vi "Qudi_ROI_multicolour_scan_Kinetix.vi"(3 "N Z positions":i32) -> ()   [LabVIEW 2015]
uses:
  <vilib>/rvi/Analysis/control/PID/Typedef/niFpgaPID_PIGains.ctl
  <vilib>/Platform/TimedLoop/XDataNode/timing_clust.ctl
  <vilib>/Platform/TimedLoop/XDataNode/nitl_modes.ctl
  <vilib>/Platform/TimedLoop/XDataNode/wakeup.ctl
  <vilib>/rvi/FXPMathLib/basic elements/FxpIntAccumulator/subVIs/nifxpmath_IntAccumulator_SimConfig.ctl
  <vilib>/rvi/Emulation/niFpgaGetClockAttributes.vi
  <vilib>/rvi/Emulation/niFpgaSctlEmulationGetInTimedLoop.vi
  <vilib>/rvi/Emulation/niFpgaEmulationReportErrorSimple.vi
  <vilib>/rvi/Emulation/niFpgaProcessEmulError.vi
  <vilib>/rvi/eio/common/nirviEmuTemplateMethod_errors.vi
  <vilib>/rvi/Analysis/common/codeGenErrors/XNode/niFpgaXNodeCodeGenErrorHandle.vi
  <vilib>/rvi/Emulation/niFpgaCriticalErrorInLSC.vi
  <vilib>/rvi/FXPMathLib/basic elements/FxpIntAccumulator/simVIs/DllFxpIntAccumulator_sub.vi
  <vilib>/rvi/Analysis/control/PID/SubVIs/niFpgaPID_PIWrapper.vi
  <vilib>/eio/EIONode/EIONode.xnode
  <vilib>/rvi/Analysis/measure/dc-rms/XNode/niFpgaDC-RMS.xnode
  <vilib>/Platform/TimedLoop/XDataNode/XDataNode.xnode
  <vilib>/rvi/FXPMathLib/basic elements/FxpIntAccumulator/XNode/nifxpmath_IntAccumulator.xnode
  <vilib>/rvi/FXPMathLib/FxpMul/XNode/nifxpmath_Multiplier.xnode
  <vilib>/Platform/TimedLoop/XDataNode/XDNodeRunTimeDep.lvlib
  <vilib>/rvi/FXPMathLib/sim/FxpSim.dll
panel:
  out "duration_ms":u32
  out "X":i16
  out "Y":i16
  out "Sum":i16
  out "counter":u32
  out "output":i16
  in  "reset":bool
  in  "reset_counter":bool
  in  "autofocus":bool
  in  "setpoint":i16
  in  "P":i16
  in  "I":i16
  in  "ref_axis":bool
  in  "integration_time_us":u32=100 caption="Count(uSec)"
  in  "exposure_time_ms":u16
  in  "stop":bool
  out "Images acquired":i32
  in  "Laser lines":i32[](array[numeric])=[0, 0, 0, 0, 0, 0, 0, 0, 0, 0]
  in  "N laser lines":i32
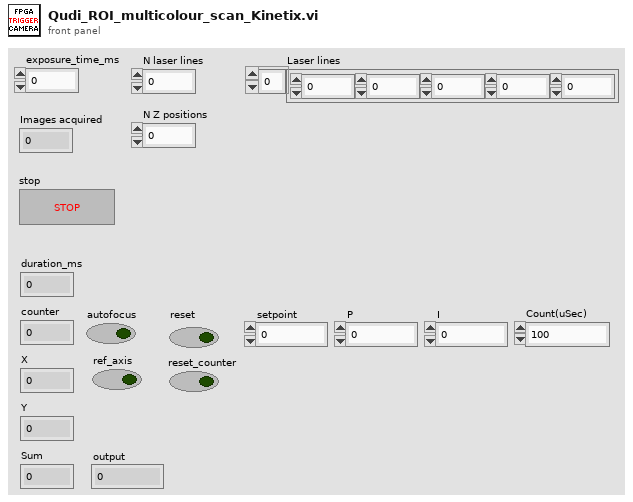
[diagram p1: front panel]
types:
  T1 = typedef "niFpgaPID_PIGains.ctl" = cluster{"proportional gain":sgl, "integral gain":sgl}
  T2 = typedef "XDNodeRunTimeDep.lvlib/timing_clust.ctl" = cluster{"Expected End [f-1]":u64, "Actual End [f-1]":u64, "Finished Late? [f-1]":bool, "Expected End [i-1]":u64, "Actual End [i-1]":u64, "Finished Late? [i-1]":bool, "Expected Start [i]":u64, "Actual Start [i]":u64, "Expected Start [f]":u64, "Actual Start [f]":u64, "Source Name":string, "Structure Name":string, "Period":i64, "Deadline":i64, "Offset":i64, "Start":i64, "Priority":i32, "Timeout":i32, "Mode":T3, "Wakeup Reason":T4, "Error":errorcluster, "Source Type":string, "Secondary Source Type":string, "Global End Time":u64, "Global Start Time":u64, "Frame Duration":u64, "Iteration Duration":u64, "Assigned CPU":i32, "I/O Scan Engine Mode":u32}
  T3 = typedef "XDNodeRunTimeDep.lvlib/nitl_modes.ctl" = enum32{"No Change", "Process missed periods, maintain original phase", "Discard missed periods, maintain original phase", "Process missed periods, ignore original phase", "Discard missed periods, ignore original phase"}
  T4 = typedef "XDNodeRunTimeDep.lvlib/wakeup.ctl" = enum32{"Normal", "Aborted", "Asynchronous wakeup", "Timing source error", "Timed loop error", "Timeout"}
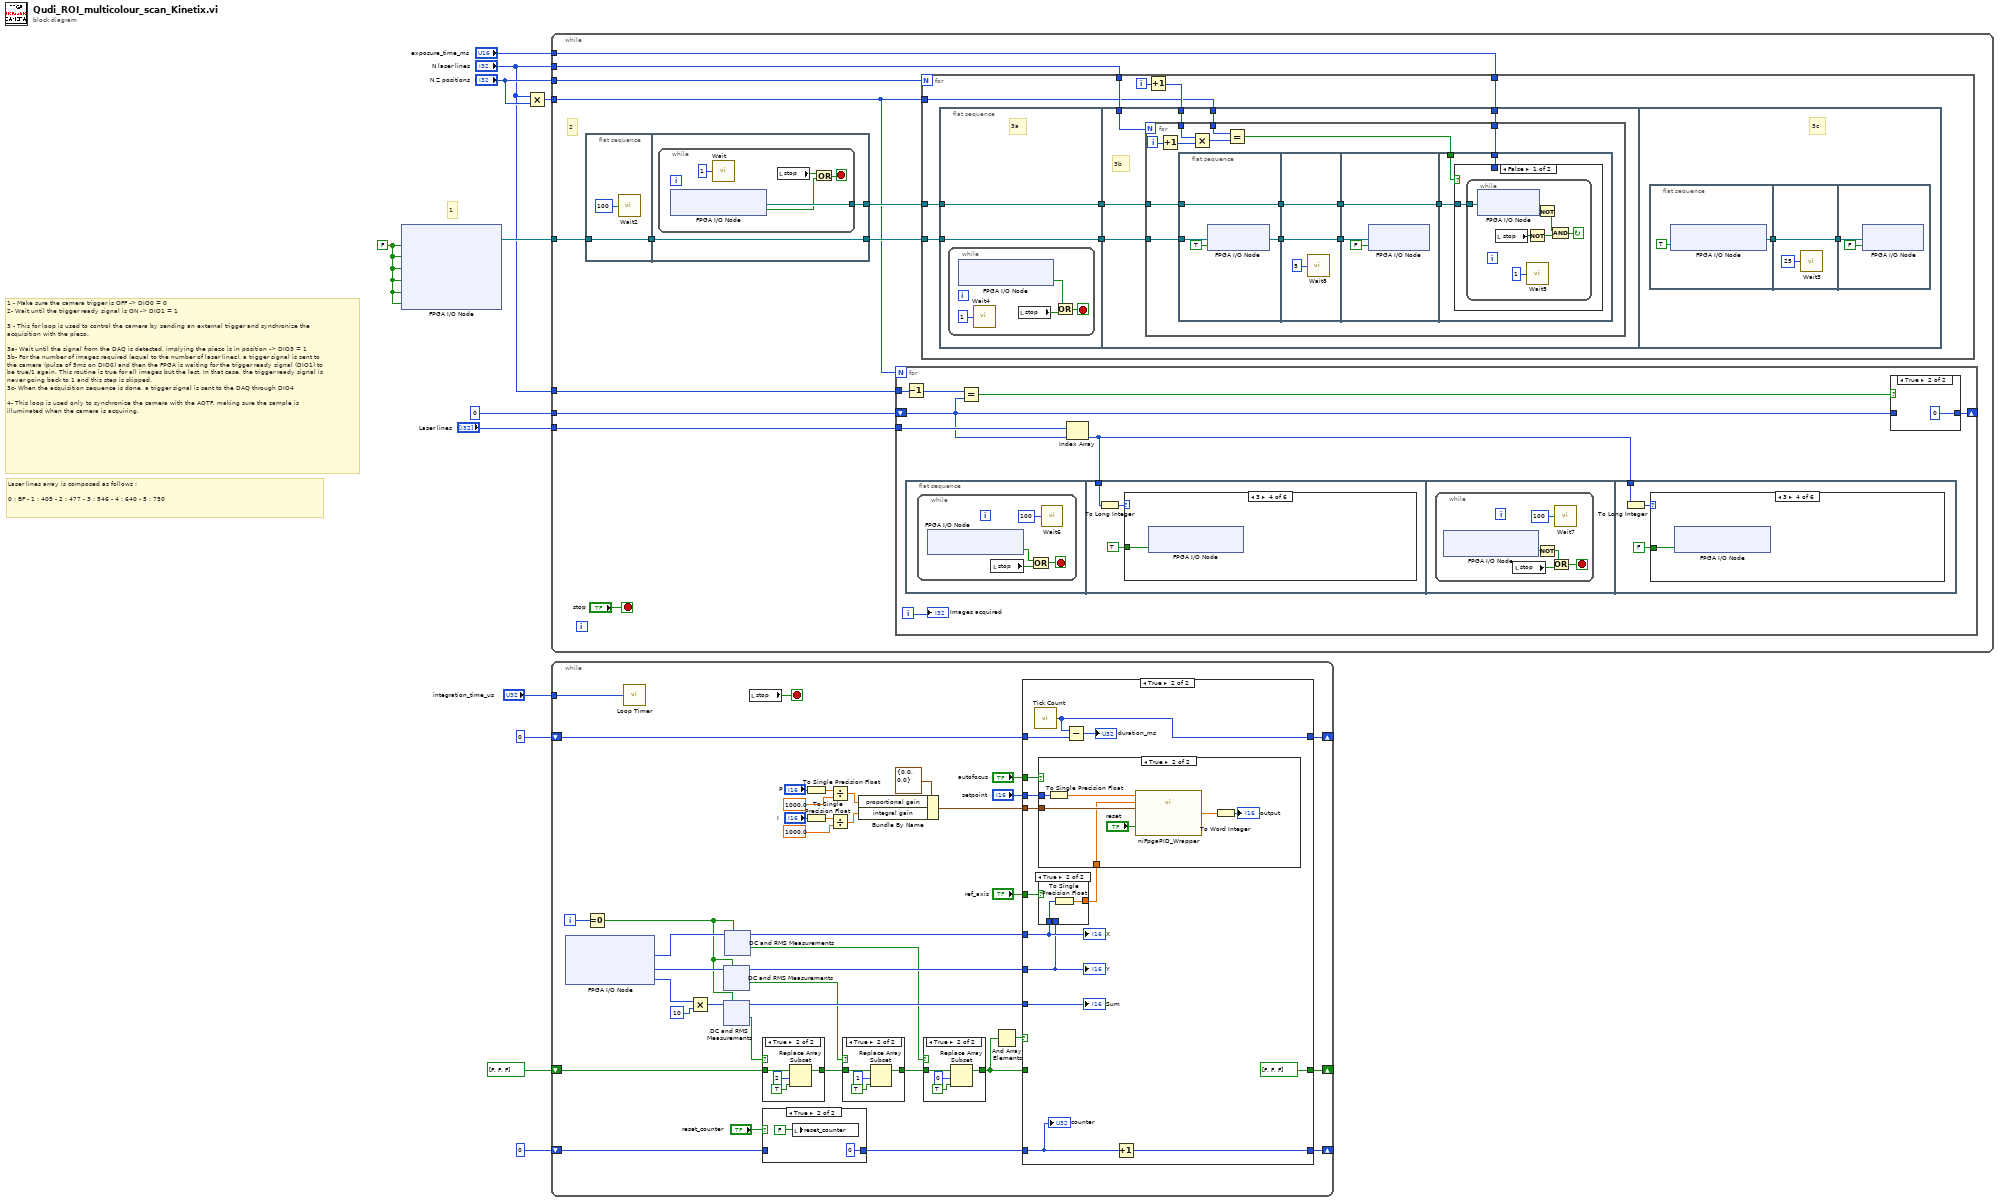
[diagram p0: block diagram]
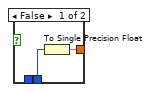
[diagram p7: hidden frame]
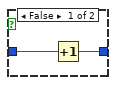
[diagram p9: hidden frame]
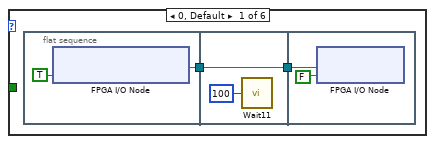
[diagram p10: hidden frame]
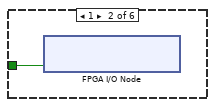
[diagram p11: hidden frame]
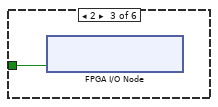
[diagram p12: hidden frame]
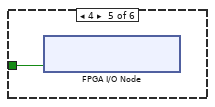
[diagram p13: hidden frame]
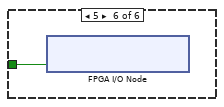
[diagram p14: hidden frame]
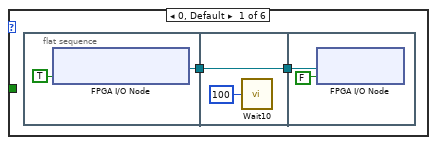
[diagram p15: hidden frame]
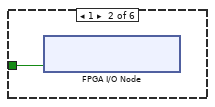
[diagram p16: hidden frame]
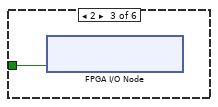
[diagram p17: hidden frame]
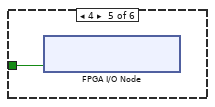
[diagram p18: hidden frame]
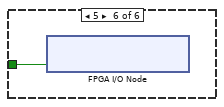
[diagram p19: hidden frame]
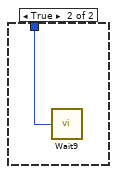
[diagram p20: hidden frame]
diagram:
  w5 = FALSE ("Connector0/DIO0")
  # "Laser lines array is composed as follows :\n\n0 : BF - 1 : 405 - 2 : 477 - 3 : 546 - 4 : 640 - 5 : 750"
  # "1"
  # "1 - Make sure the camera trigger is OFF -> DIO0 = 0\n2- Wait until the trigger ready signal is ON -> DIO1 = 1\n\n3 - This for loop is used to control the camera by sending an external trigger and synchronize the acquisition with the piezo.\n\n3a- Wait until the signal from the DAQ is detected, implying the piezo is in position -> DIO3 = 1 \n3b- For the number of images required (equal to the number of laser lines), a trigger signal is sent to the camera (pulse of 5ms on DIO0) and then the FPGA is waiting for the trigger ready signal (DIO1) to be true/1 again. This routine is true for all images but the last. In that case, the trigger ready signal is never going back to 1 and this step is skipped. \n3c- When the acquisition sequence is done, a trigger signal is sent to the DAQ through DIO4\n\n4- This loop is used only to synchronize the camera with the AOTF, making sure the sample is illuminated when the camera is acquiring."
  n1 = xnode "FPGA I/O Node"("Connector0/DIO0"=w5, "Connector0/DIO6"=w5, "Connector0/DIO7"=w5, "Connector0/DIO8"=w5, "Connector0/DIO9"=w5, "Connector0/DIO10"=w5) -> ("FPGA I/O Out"=w12:refnum<k21>)  [unwired: 6 in, 5 out]
  n2 = Multiply(x="N laser lines", y="N Z positions") -> (x*y=w8:i32)
  n3 = while {
    tunnel: w12 -> [w23]
    tunnel: "Laser lines" -> [w20]
    tunnel: 0 -> [w19]
    tunnel: "N Z positions" -> [w18]
    tunnel: "N laser lines" -> [w17]
    tunnel: w8 -> [w16]
    tunnel: "N laser lines" -> [w15]
    tunnel: "exposure_time_ms" -> [w14]
    stop <- "stop" stop-if-true
    # "2"
    n4 = flat-sequence {
      tunnel: w23 -> [w78]
      tunnel: [w78] -> w24
      tunnel: w24 -> [w80]
      tunnel: [w80] -> w22
      tunnel: [w79] -> w21
      frame #0 {
        n5 = call "Wait2"("Count(uSec)"=u8 100 ("Count(mSec)")) -> ()  [unwired: 1 out]
      }
      frame #1 {
        n6 = while {
          tunnel: [w85] -> w79
          stop <- w83 stop-if-true
          n7 = xnode "FPGA I/O Node"() -> ("Connector0/DIO1"=w81:bool, "FPGA I/O Out"=w85:refnum<k21>)  [unwired: 1 in]
          n8 = call "Wait"("Count(mSec)"=u8 1) -> ()  [unwired: 1 out]
          n9 = local read "stop"() -> (w84:bool)
          n10 = Or(x=w84, y=w81) -> (x .or. y?=w83:bool)
        }
      }
    }
    n11 = for {
      N: w16 -> [_]
      shift-right: [w30] -> _
      shift-left: w19 -> [w28]
      tunnel: w20 -> [w29]
      tunnel: w15 -> [w27]
      i -> [w25]
      n12 = Decrement(x=w27) -> (x-1=w26:i32)
      n13 = flat-sequence {
        tunnel: w32 -> [w41]
        tunnel: w32 -> [w61]
        frame #0 {
          n14 = while {
            stop <- w38 stop-if-true
            n15 = xnode "FPGA I/O Node"() -> ("Connector0/DIO2"=w39:bool)  [unwired: 1 in, 1 out]
            n16 = local read "stop"() -> (w36:bool)
            n17 = Or(x=w39, y=w36) -> (x .or. y?=w38:bool)
            n18 = call "Wait6"("Count(uSec)"=u8 100 ("Count(mSec)")) -> ()  [unwired: 1 out]
          }
        }
        frame #1 {
          n19 = To Long Integer(number=w41) -> (32bit integer=w42:i32)
          n20 = case shown="3" w42 {
            tunnel: TRUE ("Connector0/DIO6") -> [_ w51 w52 w53 w54 w55]
            frame 0, Default {
              n21 = flat-sequence {
                tunnel: [w45] -> w44
                tunnel: w44 -> [w47]
                tunnel: [w47] -> w43
                tunnel: w43 -> [w50]
                frame #0 {
                  n22 = xnode "FPGA I/O Node"("Connector0/DIO5"=TRUE) -> ("FPGA I/O Out"=w45:refnum<k21>)  [unwired: 1 in]
                }
                frame #1 {
                  n23 = call "Wait11"("Count(uSec)"=u32 100) -> ()  [unwired: 1 out]
                }
                frame #2 {
                  n24 = xnode "FPGA I/O Node"("I/O Item"=FALSE, "FPGA I/O In"=w50) -> ()  [unwired: 1 out]
                }
              }
            }
            frame 1 {
              n25 = xnode "FPGA I/O Node"("Connector0/DIO8"=w51) -> ()  [unwired: 1 in, 1 out]
            }
            frame 2 {
              n26 = xnode "FPGA I/O Node"("Connector0/DIO9"=w52) -> ()  [unwired: 1 in, 1 out]
            }
            frame 3 {
              n27 = xnode "FPGA I/O Node"("Connector0/DIO6"=w53) -> ()  [unwired: 1 in, 1 out]
            }
            frame 4 {
              n28 = xnode "FPGA I/O Node"("Connector0/DIO7"=w54) -> ()  [unwired: 1 in, 1 out]
            }
            frame 5 {
              n29 = xnode "FPGA I/O Node"("Connector0/DIO10"=w55) -> ()  [unwired: 1 in, 1 out]
            }
          }
        }
        frame #2 {
          n30 = while {
            stop <- w58 stop-if-true
            n31 = xnode "FPGA I/O Node"() -> ("Connector0/DIO2"=w59:bool)  [unwired: 1 in, 1 out]
            n32 = local read "stop"() -> (w60:bool)
            n33 = Not(x=w59) -> (.not. x?=w56:bool)
            n34 = Or(x=w56, y=w60) -> (x .or. y?=w58:bool)
            n35 = call "Wait7"("Count(uSec)"=u8 100 ("Count(mSec)")) -> ()  [unwired: 1 out]
          }
        }
        frame #3 {
          n36 = To Long Integer(number=w61) -> (32bit integer=w62:i32)
          n37 = case shown="3" w62 {
            tunnel: FALSE ("Connector0/DIO6") -> [_ w72 w73 w74 w75 w76]
            frame 0, Default {
              n38 = flat-sequence {
                tunnel: [w66] -> w65
                tunnel: w65 -> [w68]
                tunnel: [w68] -> w64
                tunnel: w64 -> [w71]
                frame #0 {
                  n39 = xnode "FPGA I/O Node"("Connector0/DIO5"=TRUE) -> ("FPGA I/O Out"=w66:refnum<k21>)  [unwired: 1 in]
                }
                frame #1 {
                  n40 = call "Wait10"("Count(uSec)"=u32 100) -> ()  [unwired: 1 out]
                }
                frame #2 {
                  n41 = xnode "FPGA I/O Node"("I/O Item"=FALSE, "FPGA I/O In"=w71) -> ()  [unwired: 1 out]
                }
              }
            }
            frame 1 {
              n42 = xnode "FPGA I/O Node"("Connector0/DIO8"=w72) -> ()  [unwired: 1 in, 1 out]
            }
            frame 2 {
              n43 = xnode "FPGA I/O Node"("Connector0/DIO9"=w73) -> ()  [unwired: 1 in, 1 out]
            }
            frame 3 {
              n44 = xnode "FPGA I/O Node"("Connector0/DIO6"=w74) -> ()  [unwired: 1 in, 1 out]
            }
            frame 4 {
              n45 = xnode "FPGA I/O Node"("Connector0/DIO7"=w75) -> ()  [unwired: 1 in, 1 out]
            }
            frame 5 {
              n46 = xnode "FPGA I/O Node"("Connector0/DIO10"=w76) -> ()  [unwired: 1 in, 1 out]
            }
          }
        }
      }
      n47 = Equal?(x=w26, y=w28) -> (x = y?=w31:bool)
      n48 = Index Array(array=w29, index=w28) -> (element=w32:i32)
      n49 = case shown="True" w31 {
        tunnel: w28 -> [w34 _]
        tunnel: [w33 0] -> w30
        frame False {
          n50 = Increment(x=w34) -> (x+1=w33:i32)
        }
        frame True {
        }
      }
      "Images acquired" <- w25
    }
    n51 = for {
      N: w18 -> [_]
      tunnel: w22 -> [w93]
      tunnel: w21 -> [w94]
      tunnel: w17 -> [w89]
      tunnel: w16 -> [w87]
      tunnel: w14 -> [w86]
      i -> [w90]
      n52 = flat-sequence {
        tunnel: w93 -> [w95]
        tunnel: w94 -> [w96]
        tunnel: [w96] -> w92
        tunnel: [w95] -> w91
        tunnel: w92 -> [w106]
        tunnel: w91 -> [w105]
        tunnel: w89 -> [w104]
        tunnel: w88 -> [w103]
        tunnel: w87 -> [w102]
        tunnel: w86 -> [w101]
        frame #0 {
          # "3a"
          n53 = while {
            stop <- w98 stop-if-true
            n54 = xnode "FPGA I/O Node"() -> ("Connector0/DIO3"=w99:bool)  [unwired: 1 in, 1 out]
            n55 = call "Wait4"("Count(mSec)"=u8 1) -> ()  [unwired: 1 out]
            n56 = local read "stop"() -> (w100:bool)
            n57 = Or(x=w99, y=w100) -> (x .or. y?=w98:bool)
          }
        }
        frame #1 {
          # "3b"
          n58 = for {
            N: w104 -> [_]
            tunnel: w106 -> [w115]
            tunnel: w105 -> [w114]
            tunnel: w103 -> [w111]
            tunnel: w102 -> [w109]
            tunnel: w101 -> [w107]
            i -> [w113]
            n59 = Increment(x=w113) -> (x+1=w112:i32)
            n60 = flat-sequence {
              tunnel: [w123] -> w120
              tunnel: [w121] -> w119
              tunnel: w114 -> [w122]
              tunnel: w115 -> [w121]
              tunnel: w120 -> [w127]
              tunnel: [w127] -> w118
              tunnel: [w126] -> w117
              tunnel: w119 -> [w126]
              tunnel: w118 -> [w129]
              tunnel: [w128] -> w116
              tunnel: w117 -> [w128]
              tunnel: w116 -> [w133]
              tunnel: w108 -> [w132]
              tunnel: w107 -> [w131]
              frame #0 {
                n61 = xnode "FPGA I/O Node"("I/O Item"=TRUE ("Connector0/DIO0"), "FPGA I/O In"=w122) -> ("FPGA I/O Out"=w123:refnum<k21>)
              }
              frame #1 {
                n62 = call "Wait8"("Count(mSec)"=u8 5) -> ()  [unwired: 1 out]
              }
              frame #2 {
                n63 = xnode "FPGA I/O Node"("I/O Item"=FALSE ("Connector0/DIO0"), "FPGA I/O In"=w129) -> ()  [unwired: 1 out]
              }
              frame #3 {
                n64 = case shown="False" w132 {
                  tunnel: w133 -> [w134 _]
                  tunnel: w131 -> [_ w142]
                  frame False {
                    n65 = while {
                      tunnel: w134 -> [w141]
                      stop <- w137 continue-if-true
                      n66 = xnode "FPGA I/O Node"("FPGA I/O In"=w141) -> ("I/O Item"=w138:bool)  [unwired: 1 out]
                      n67 = local read "stop"() -> (w140:bool)
                      n68 = Not(x=w140) -> (.not. x?=w139:bool)
                      n69 = call "Wait5"("Count(mSec)"=u8 1) -> ()  [unwired: 1 out]
                      n70 = Not(x=w138) -> (.not. x?=w135:bool)
                      n71 = And(x=w135, y=w139) -> (x .and. y?=w137:bool)
                    }
                  }
                  frame True {
                    n72 = call "Wait9"("Count(mSec)"=w142) -> ()  [unwired: 1 out]
                  }
                }
              }
            }
            n73 = Multiply(x=w111, y=w112) -> (x*y=w110:i32)
            n74 = Equal?(x=w109, y=w110) -> (x = y?=w108:bool)
          }
        }
        frame #2 {
          # "3c"
          n75 = flat-sequence {
            tunnel: [w146] -> w144
            tunnel: w144 -> [w147]
            tunnel: [w147] -> w143
            tunnel: w143 -> [w149]
            frame #0 {
              n76 = xnode "FPGA I/O Node"("Connector0/DIO4"=TRUE) -> ("FPGA I/O Out"=w146:refnum<k21>)  [unwired: 1 in]
            }
            frame #1 {
              n77 = call "Wait3"("Count(mSec)"=u8 25) -> ()  [unwired: 1 out]
            }
            frame #2 {
              n78 = xnode "FPGA I/O Node"("I/O Item"=FALSE ("Connector0/DIO0"), "FPGA I/O In"=w149) -> ()  [unwired: 1 out]
            }
          }
        }
      }
      n79 = Increment(x=w90) -> (x+1=w88:i32)
    }
  }
  n80 = while {
    shift-right: [w175] -> _
    shift-left: bool[] [FALSE, FALSE, FALSE] ("initialized array") -> [w183]
    shift-right: [w173] -> _
    shift-left: u32 0 -> [w174]
    tunnel: "integration_time_us" -> [w172]
    shift-right: [w171] -> _
    shift-left: u32 0 -> [w169]
    i -> [w189]
    stop <- w151 stop-if-true
    n81 = xnode "FPGA I/O Node"() -> ("Connector0/AI0"=w190:i16, "Connector0/AI1"=w187:i16, "Connector0/AI2"=w154:i16)  [unwired: 3 in, 3 out]
    n82 = Equal To 0?(x=w189) -> (x = 0?=w184:bool)
    n83 = call "Loop Timer"("Count(uSec)"=w172) -> ()  [unwired: 1 out]
    n84 = Multiply(x=w154, y=i16 10) -> (x*y=w153:i16)
    n85 = xnode "DC and RMS Measurements"("input data"=w187, "reset"=w184) -> ("DC"=w186:i16, "output valid"=w179:bool)
    n86 = xnode "DC and RMS Measurements"("input data"=w153, "reset"=w184) -> ("DC"=w185:i16, "output valid"=w180:bool)
    n87 = xnode "DC and RMS Measurements"("input data"=w190, "reset"=w184) -> ("DC"=w188:i16, "output valid"=w178:bool)
    n88 = local read "stop"() -> (w151:bool)
    n89 = case shown="True" w180 {
      tunnel: w183 -> [w199 w202]
      tunnel: [w199 w200] -> w182
      frame False {
      }
      frame True {
        n90 = Replace Array Subset(array=w202, new element=TRUE, index=2) -> (w200:bool[])
      }
    }
    n91 = case shown="True" "reset_counter" {
      tunnel: w169 -> [w191 _]
      tunnel: [w191 u32 0] -> w168
      frame False {
      }
      frame True {
        n92 = local write "reset_counter"(FALSE ("Reset counter")) -> ()
      }
    }
    n93 = To Single Precision Float(number="P") -> (single precision float=w161:sgl)
    n94 = To Single Precision Float(number="I") -> (single precision float=w158:sgl)
    n95 = Divide(x=w161, y=sgl 1000.0) -> (x/y=w159:sgl)
    n96 = Divide(x=w158, y=sgl 1000.0) -> (x/y=w156:sgl)
    n97 = case shown="True" w179 {
      tunnel: w182 -> [w204 w207]
      tunnel: [w204 w205] -> w181
      frame False {
      }
      frame True {
        n98 = Replace Array Subset(array=w207, new element=TRUE, index=1) -> (w205:bool[])
      }
    }
    n99 = Bundle By Name(cluster=T1 {"proportional gain"=0.0, "integral gain"=0.0} ("gains"), "proportional gain"=w159, "integral gain"=w156) -> (w162:T1)
    n100 = case shown="True" w178 {
      tunnel: [w194 w196] -> w176
      tunnel: w181 -> [w194 w195]
      frame False {
      }
      frame True {
        n101 = Replace Array Subset(array=w195, new element=TRUE, index=0) -> (w196:bool[])
      }
    }
    n102 = And Array Elements(Boolean array=w176) -> (logical AND=w177:bool)
    n103 = case shown="True" w177 {
      tunnel: w188 -> [_ w214]
      tunnel: w186 -> [_ w212]
      tunnel: w185 -> [_ w220]
      tunnel: w176 -> [w211 _]
      tunnel: [w211 bool[] [FALSE, FALSE, FALSE] ("initialized array")] -> w175
      tunnel: w174 -> [w210 w224]
      tunnel: [w210 w222] -> w173
      tunnel: w168 -> [w209 w219]
      tunnel: [w209 w221] -> w171
      tunnel: "autofocus" -> [_ w218]
      tunnel: "setpoint" -> [_ w217]
      tunnel: w162 -> [_ w216]
      tunnel: "ref_axis" -> [_ w215]
      frame False {
      }
      frame True {
        n104 = call "Tick Count"() -> ("Tick Count(mSec)"=w222:u32)
        n105 = case shown="True" w215 {
          tunnel: w214 -> [_ w229]
          tunnel: [w226 w228] -> w213
          tunnel: w212 -> [w227 _]
          frame False {
            n106 = To Single Precision Float(number=w227) -> (single precision float=w226:sgl)
          }
          frame True {
            n107 = To Single Precision Float(number=w229) -> (single precision float=w228:sgl)
          }
        }
        n108 = case shown="True" w218 {
          tunnel: w217 -> [_ w236]
          tunnel: w216 -> [_ w234]
          tunnel: w213 -> [_ w230]
          frame False {
          }
          frame True {
            n109 = To Single Precision Float(number=w236) -> (single precision float=w235:sgl)
            n110 = call-poly <vilib>:"niFpgaPID_Wrapper.vi"("setpoint"=w235, "reset? (F)"="reset", "process variable"=w230, "gains"=w234) -> ("output"=w232:sgl)  [unwired: 9 in, 2 out]
            n111 = To Word Integer(number=w232) -> (16bit integer=→"output":i16)
          }
        }
        n112 = Subtract(x=w222, y=w224) -> (x-y=→"duration_ms":u32)
        n113 = Increment(x=w219) -> (x+1=w221:u32)
        "X" <- w214
        "Y" <- w212
        "Sum" <- w220
        "counter" <- w219
      }
    }
  }
